vi "AssertIndexValue.vi"(0 "VI Reference In":refnum<vi>, 1 "Test Label":string, 2 "delimiter (>>)":string=">>", 3 "Assert Only? (F)":bool, 5 "Control Path":string, 7 "Row Index":i32, 9 "Item Value":string, 11 "Error In":errorcluster, 12 "Assert Interval(10 ms)":u32=10, 13 "Timeout(5 sec)":dbl=5.0, 14 "Column Index":i32) -> (4 "VI Reference Out":refnum<vi>, 6 "Asserted Value":string, 15 "Error Out":errorcluster)   [LabVIEW 2016, in "Drona.lvlib" / "AssertControlValue.lvlib" / "AssertMCListbox.lvlib"]
doc: "Asserts if the item name on specified index in the multi-column listbox control is equal.\n\nThe input control name is given as a string, incase of the path, use delimiters in between the path.\nThis VI gets the control value until the value is equal to the input value."
uses:
  AssertMCListbox.lvlib
  Get/GetControlRef/GetControlRefByPath.vi
  <vilib>/Utility/error.llb/Error Cluster From Error Code.vi
  <vilib>/addons/_JKI Toolkits/Caraya/classes/Assert/Assert Equal Value_Variant.vi
  <vilib>/ErrorRing/Error Ring.xnode
  <vilib>/addons/_JKI Toolkits/Caraya/classes/Assert/Assert.lvclass
  Get/GetControlRef/GetControlRef.lvlib
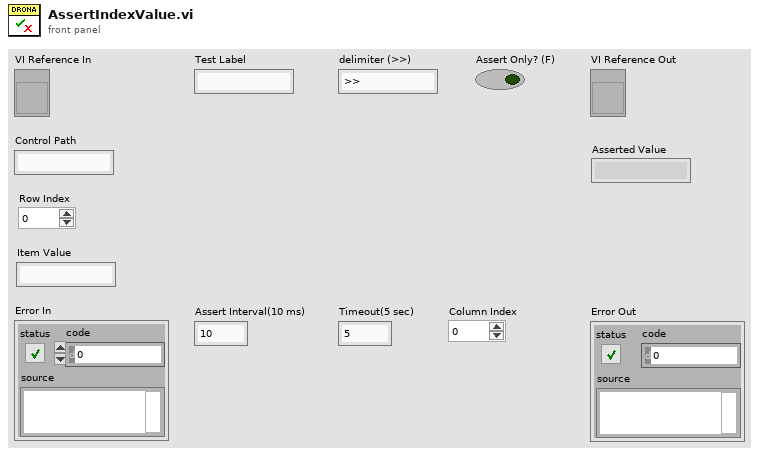
[diagram p1: front panel]
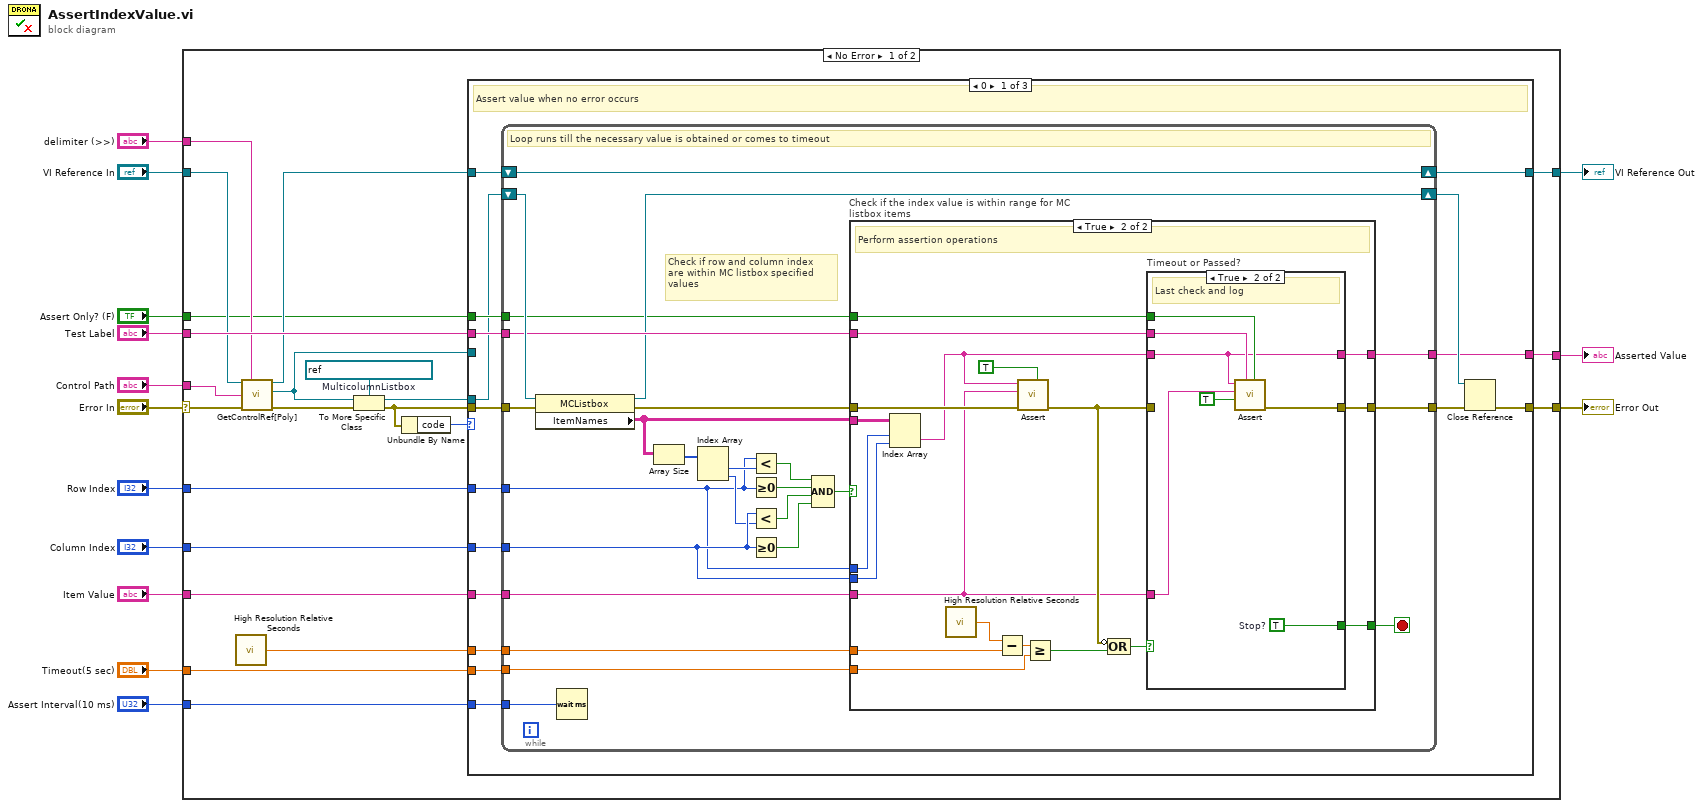
[diagram p0: block diagram]
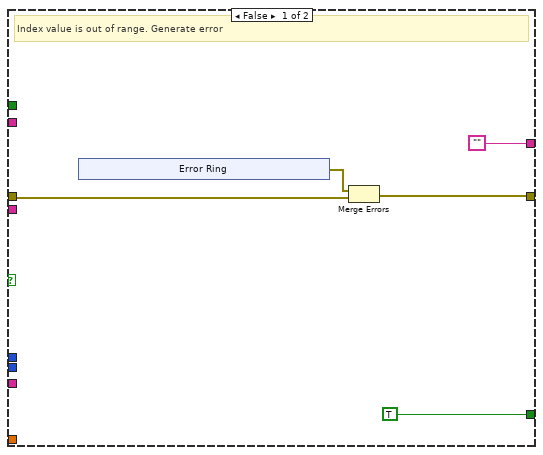
[diagram p2: hidden frame]
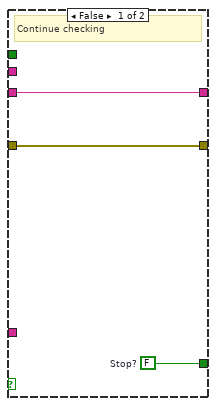
[diagram p3: hidden frame]
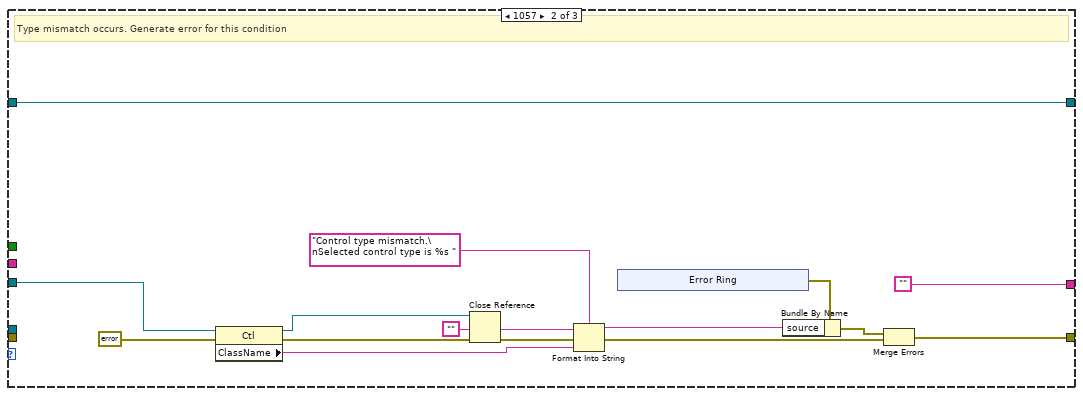
[diagram p4: hidden frame]
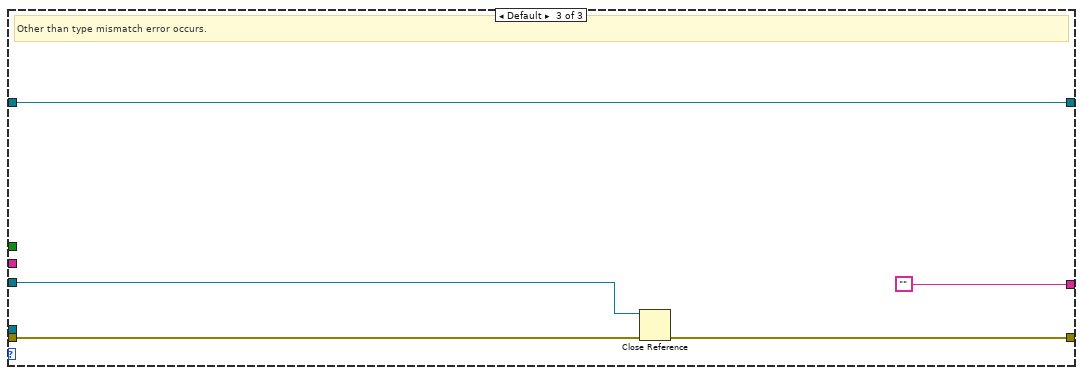
[diagram p5: hidden frame]
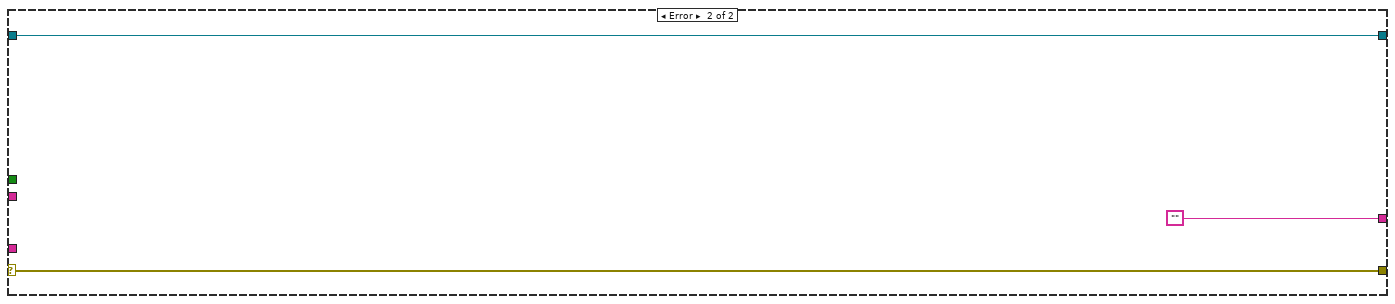
[diagram p6: hidden frame]
diagram:
  n1 = case shown="No Error" "Error In" {
    selector: "Error In" -> [w31 w144]
    tunnel: "Timeout(5 sec)" -> [w36 _]
    tunnel: [w35 w143] -> w13
    tunnel: "Row Index" -> [w34 _]
    tunnel: [w25 w144] -> w12
    tunnel: "Assert Interval(10 ms)" -> [w33 _]
    tunnel: "Test Label" -> [w32 _]
    tunnel: "VI Reference In" -> [w30 w143]
    tunnel: "Control Path" -> [w29 _]
    tunnel: "delimiter (>>)" -> [w24 _]
    tunnel: "Assert Only? (F)" -> [w23 _]
    tunnel: [w22 ""] -> w2
    tunnel: "Item Value" -> [w19 _]
    tunnel: "Column Index" -> [w15 _]
    frame No Error {
      w21 = refnum<vi> refnum  # MulticolumnListbox
      n2 = call <vilib>:"High Resolution Relative Seconds.vi"() -> ("relative seconds"=w28:dbl)
      n3 = call-poly "GetControlRef[Poly].vi"("VI Reference In"=w30, "delimiter (>>)"=w24, "Control Path"=w29, "error In"=w31) -> ("VI Reference Out"=w26:refnum<vi>, "Ctl Refnum"=w16:refnum<vi>, "error out"=w27:errorcluster)  [unwired: 9 in]
      n4 = To More Specific Class(target class=w21, reference=w16, error in=w27) -> (specific class reference=w20:refnum<vi>, error out=w18:errorcluster)
      n5 = Unbundle By Name(w18) -> ("code"=w17:i32)
      n6 = case shown="0" w17 {
        tunnel: w36 -> [w52 _ _]
        tunnel: [w51 w130 w141] -> w35
        tunnel: w34 -> [w50 _ _]
        tunnel: w33 -> [w48 _ _]
        tunnel: w32 -> [w47 _ _]
        tunnel: w28 -> [w46 _ _]
        tunnel: w26 -> [w45 w130 w141]
        tunnel: [w44 w118 w138] -> w25
        tunnel: w23 -> [w42 _ _]
        tunnel: [w41 "" ""] -> w22
        tunnel: w18 -> [w40 _ w140]
        tunnel: w20 -> [w39 _ _]
        tunnel: w19 -> [w38 _ _]
        tunnel: w16 -> [_ w117 w137]
        tunnel: w15 -> [w37 _ _]
        frame 0 {
          # "Assert value when no error occurs"
          n7 = while {
            tunnel: w50 -> [w53]
            tunnel: w52 -> [w76]
            tunnel: w46 -> [w77]
            tunnel: w40 -> [w71]
            tunnel: [w74] -> w49
            tunnel: w48 -> [w72]
            tunnel: w47 -> [w68]
            shift-right: [w69] -> w51
            shift-left: w45 -> [w69]
            shift-right: [w67] -> w43
            shift-left: w39 -> [w70]
            tunnel: w42 -> [w66]
            tunnel: [w65] -> w41
            tunnel: w38 -> [w64]
            tunnel: w37 -> [w58]
            stop <- w75 stop-if-true
            # "Check if row and column index \nare within MC listbox specified \nvalues"
            # "Loop runs till the necessary value is obtained or comes to timeout"
            n8 = property on="Property Node" class="MCListbox"(reference=w70, error in=w71) -> (reference out=w67:refnum<vi>, error out=w73:errorcluster, "ItemNames"=w57:string[][])
            n9 = Wait (ms)(milliseconds to wait=w72) -> ()  [unwired: 1 out]
            n10 = Array Size(array=w57) -> (size(s)=w56:i32[])
            n11 = Index Array(array=w56) -> (element #1=w55:i32, element #2=w54:i32)  [unwired: 2 in]
            n12 = Less?(x=w53, y=w55) -> (x < y?=w63:bool)
            n13 = Greater Or Equal To 0?(x=w53) -> (x >= 0?=w62:bool)
            n14 = Less?(x=w58, y=w54) -> (x < y?=w61:bool)
            n15 = Greater Or Equal To 0?(x=w58) -> (x >= 0?=w60:bool)
            n16 = Compound Arithmetic op=AND(w63, w62, w61, w60) -> (w59:bool)
            n17 = case "Check if the index value is within range for MC listbox items" shown="True" w59 {
              tunnel: w77 -> [_ w106]
              tunnel: w76 -> [_ w103]
              tunnel: [TRUE w95] -> w75
              tunnel: [w78 w96] -> w74
              tunnel: w68 -> [_ w101]
              tunnel: w66 -> [_ w94]
              tunnel: ["" w93] -> w65
              tunnel: w64 -> [_ w92]
              tunnel: w57 -> [_ w91]
              tunnel: w73 -> [w79 w102]
              tunnel: w58 -> [_ w89]
              tunnel: w53 -> [_ w88]
              frame False {
                # "Index value is out of range. Generate error"
                n18 = xnode "Error Ring"() -> ("error out"=w80:errorcluster)
                n19 = Merge Errors(w80, w79) -> (w78:errorcluster)
              }
              frame True {
                # "Perform assertion operations"
                n20 = Index Array(array=w91, index (row)=w88, index (col)=w89) -> (element=w90:string)
                n21 = call <vilib>:"High Resolution Relative Seconds.vi"() -> ("relative seconds"=w105:dbl)
                n22 = Subtract(x=w105, y=w106) -> (x-y=w104:dbl)
                n23 = call-poly <vilib>:"Assert.vi"("Assert Only? (F)"=TRUE, "error in (no error)"=w102, "Y"=w92, "X"=w90) -> ("error out"=w99:errorcluster)  [unwired: 6 in, 1 out]
                n24 = Greater Or Equal?(x=w104, y=w103) -> (x >= y?=w100:bool)
                n25 = Compound Arithmetic op=OR(invert w99, w100) -> (w98:bool)
                n26 = case "Timeout or Passed?" shown="True" w98 {
                  tunnel: w99 -> [w109 _]
                  tunnel: w92 -> [_ w115]
                  tunnel: w90 -> [w107 w110]
                  tunnel: w101 -> [_ w116]
                  tunnel: [w109 w114] -> w96
                  tunnel: [w108 w113] -> w95
                  tunnel: w94 -> [_ w111]
                  tunnel: [w107 w110] -> w93
                  frame False {
                    w108 = FALSE  # Stop?
                    # "Continue checking"
                  }
                  frame True {
                    w113 = TRUE  # Stop?
                    # "Last check and log"
                    n27 = call-poly <vilib>:"Assert.vi"("Assert Only? (F)"=w111, "Label"=w116, "Register with caller test (F)"=TRUE, "Y"=w115, "X"=w110) -> ("error out"=w114:errorcluster)  [unwired: 5 in, 1 out]
                  }
                }
              }
            }
          }
          n28 = Close Reference(reference=w43, error in (no error)=w49) -> (error out=w44:errorcluster)
        }
        frame 1057 {
          # "Type mismatch occurs. Generate error for this condition"
          n29 = property class="Ctl"(reference=w117, error in=errorcluster {"status"=FALSE, "code"=0, "source"=""} ("error out")) -> (reference out=w119:refnum<vi>, error out=w129:errorcluster, "ClassName"=w126:string)
          n30 = Close Reference(reference=w119, error in (no error)=w129) -> (error out=w120:errorcluster)
          n31 = Format Into String(format string="Control type mismatch.\nSelected control type is %s ", initial string="", error in=w120, w126) -> (resulting string=w123:string, error out=w121:errorcluster)
          n32 = xnode "Error Ring"() -> ("error out"=w124:errorcluster)
          n33 = Bundle By Name(cluster=w124, "source"=w123) -> (w122:errorcluster)
          n34 = Merge Errors(w122, w121) -> (w118:errorcluster)
        }
        frame Default {
          # "Other than type mismatch error occurs."
          n35 = Close Reference(reference=w137, error in (no error)=w140) -> (error out=w138:errorcluster)
        }
      }
    }
    frame Error {
    }
  }
  "Error Out" <- w12
  "VI Reference Out" <- w13
  "Asserted Value" <- w2
